vi "ForceSpect.vi"(3 "Force Input":dbl, 4 "Force Tolerance":dbl, 5 "Force  Spect":dbl) -> (0 "Force Color":u32, 2 "Force OK":bool)   [LabVIEW 2017]
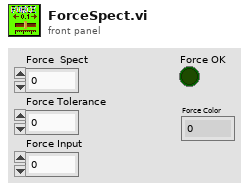
[diagram p1: front panel]
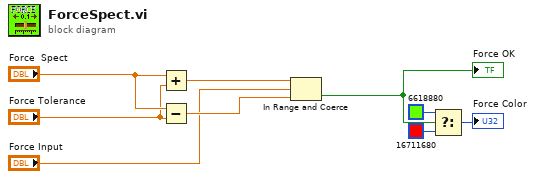
[diagram p0: block diagram]
diagram:
  n1 = Add(x="Force  Spect", y="Force Tolerance") -> (x+y=w7:dbl)
  n2 = Subtract(x="Force  Spect", y="Force Tolerance") -> (x-y=w6:dbl)
  n3 = In Range and Coerce(upper limit=w7, x="Force Input", lower limit=w6) -> (In Range?=w1:bool)  [unwired: 1 out]
  "Force OK" <- w1
  n4 = Select(t=u32 6618880, s=w1, f=u32 16711680) -> (s? t:f=→"Force Color":u32)
